vi "CreateIfNotExistsString.vi"(10 "Items":string[](array[string])=["C1", "C2", "C3"], 11 "Table Name":string="temp") -> (3 "Create If Not Existed String":string)   [LabVIEW 2015, in "DBToolkit.lvlib"]
uses:
  DBToolkit.lvlib
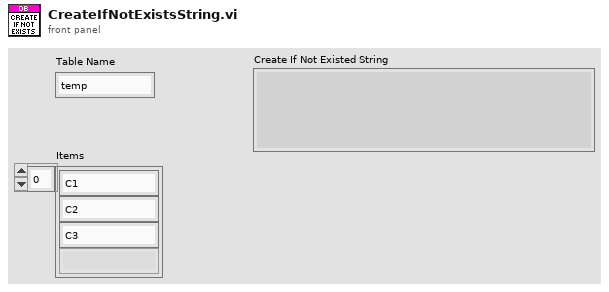
[diagram p1: front panel]
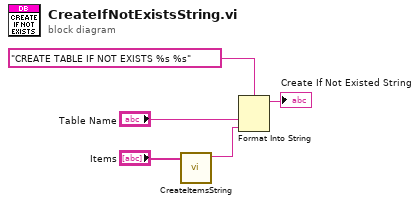
[diagram p0: block diagram]
diagram:
  n1 = call "CreateItemsString.vi"("Items"="Items") -> ("Items for CREATE"=w2:string)  [unwired: 8 in, 2 out]
  n2 = Format Into String(format string="CREATE TABLE IF NOT EXISTS %s %s", "Table Name", w2) -> (resulting string=→"Create If Not Existed String":string)  [unwired: 2 in, 1 out]
